vi "Globals.vi"() -> ()   [LabVIEW 2022 SP3]
uses:
  move_dir_lr.ctl
panel:
  in  "Direction":T1
  in  "Shift_V":i16
  in  "Shift_H":i16
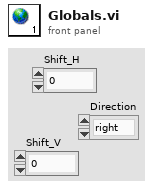
[diagram p1: front panel]
types:
  T1 = typedef "move_dir_lr.ctl" = enum16{"right", "left"}
diagram:
